vi "Extend pulse duration.vi"(10 "duration (ticks)":u32, 11 "Boolean":bool) -> (3 "out":bool)   [LabVIEW 2019, in "FPGA Utility.lvlib"]
uses:
  FPGA Utility.lvlib
  <instrlib>/_niInstr/Basic Elements/v1/FPGA/Private/Count Up U32.vi
  <instrlib>/_niInstr/Basic Elements/v1/FPGA/niInstr Basic Elements v1 FPGA.lvlib
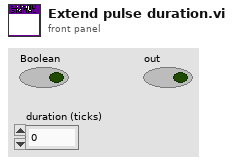
[diagram p1: front panel]
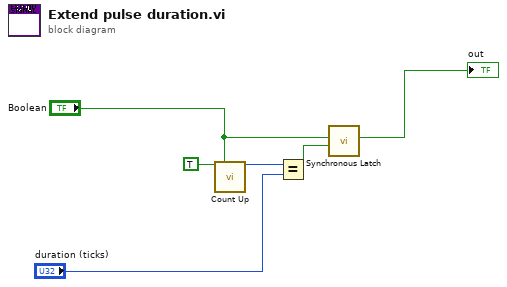
[diagram p0: block diagram]
diagram:
  n1 = call-poly <instrlib>:"Count Up.vi"("increment"=TRUE, "reset"="Boolean") -> ("count out"=w5:u32)  [unwired: 13 in]
  n2 = Equal?(x=w5, y="duration (ticks)") -> (x = y?=w3:bool)
  n3 = call <instrlib>:"Synchronous Latch.vi"("clear"=w3, "set"="Boolean") -> ("out"=→"out":bool)  [unwired: 9 in]
